vi "tester.vi"() -> ()   [LabVIEW 2014]
uses:
  <vilib>/Utility/inputDevices.llb/closeKeyboard.vi
  <vilib>/Utility/inputDevices.llb/keyboardAcquire.vi
panel:
  in  "stop":bool
  in  "SnakeLeght":i32=5
  out "Real 2D Array":u32[][](array[numeric])
  in  "FieldSizeY":i32=15
  in  "FieldSizeX":i32=10
  out "SnakeWorld":bool[][](array[boolean])
  in  "StartPointY":i32=5
  in  "StartPointX":i32=5
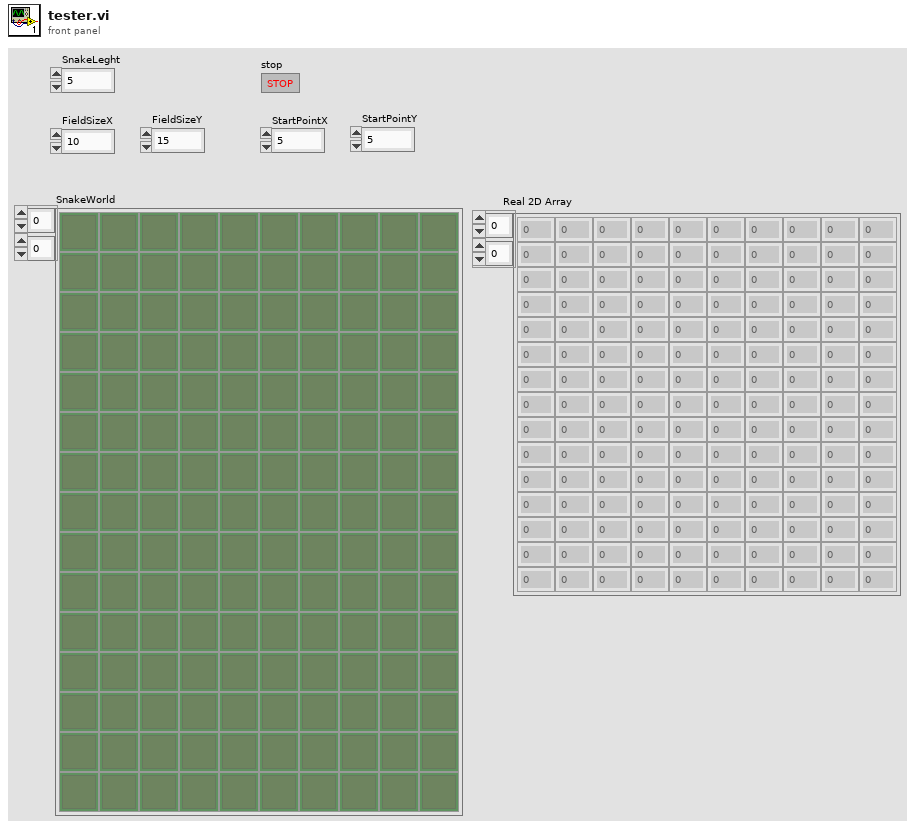
[diagram p1: front panel]
types:
  T1 = enum16{"0", "1", "2", "3", "4", "5", "6", "7", "8", "9", "A", "B", "C", "D", "E", "F", "G", "H", "I", "J", "K", "L", "M", "N", "O", "P", "Q", "R", "S", "T", "U", "V", "W", "X", "Y", "Z", "F1", "F2", "F3", "F4", "F5", "F6", "F7", "F8", "F9", "F10", "F11", "F12", "F13", "F14", "F15", "ADD", "BACK", "BACKSLASH", "CAPITAL", "COMMA", "DECIMAL", "DELETE", "DIVIDE", "DOWN", "END", "EQUALS", "ESCAPE", "GRAVE (`)", "HOME", "INSERT", "LBRACKET", "LCONTROL", "LEFT", "L ALT", "LSHIFT", "LWIN", "MINUS", "MULTIPLY", "NEXT", "NUMLOCK", "NUMPAD_0", "NUMPAD_1", "NUMPAD_2", "NUMPAD_3", "NUMPAD_4", "NUMPAD_5", "NUMPAD_6", "NUMPAD_7", "NUMPAD_8", "NUMPAD_9", "PAUSE", "PERIOD", "PRIOR (PG UP)", "RBRACKET", "RCONTROL", "RETURN", "RIGHT", "R ALT", "RSHIFT", "RWIN", "SCROLL", "SEMICOLON", "SLASH", "SPACE", "SUBTRACT", "TAB", "UP", "ENTER (num pad)", "' (quote)"}
  T2 = enum16{"0", "1", "2", "3", "4", "5", "6", "7", "8", "9", "A", "B", "C", "D", "E", "F", "G", "H", "I", "J", "K", "L", "M", "N", "O", "P", "Q", "R", "S", "T", "U", "V", "W", "X", "Y", "Z", "F1", "F2", "F3", "F4", "F5", "F6", "F7", "F8", "F9", "F10", "F11", "F12", "F13", "F14", "F15", "ADD", "BACK", "BACKSLASH", "CAPITAL", "COMMA", "DECIMAL", "DELETE", "DIVIDE", "DOWN", "END", "EQUALS", "ESCAPE", "GRAVE (`)", "HOME", "INSERT", "LBRACKET", "LCONTROL", "LEFT", "L ALT", "LSHIFT", "LWIN", "MINUS", "MULTIPLY", "NEXT", "NUMLOCK", "NUMPAD_0", "NUMPAD_1", "NUMPAD_2", "NUMPAD_3", "NUMPAD_4", "NUMPAD_5", "NUMPAD_6", "NUMPAD_7", "NUMPAD_8", "NUMPAD_9", "PAUSE", "PERIOD", "PRIOR (PG UP)", "RBRACKET", "RCONTROL", "RETURN", "RIGHT", "R ALT", "RSHIFT", "RWIN", "SCROLL", "SEMICOLON", "SLASH", "SPACE", "SUBTRACT", "TAB", "UP", "ENTER (num pad)", "' (quote)"}[]
  T3 = typedef "SnakeMovements.ctl" = enum16{"STOP", "UP", "DOWN", "RIGHT", "LEFT"}
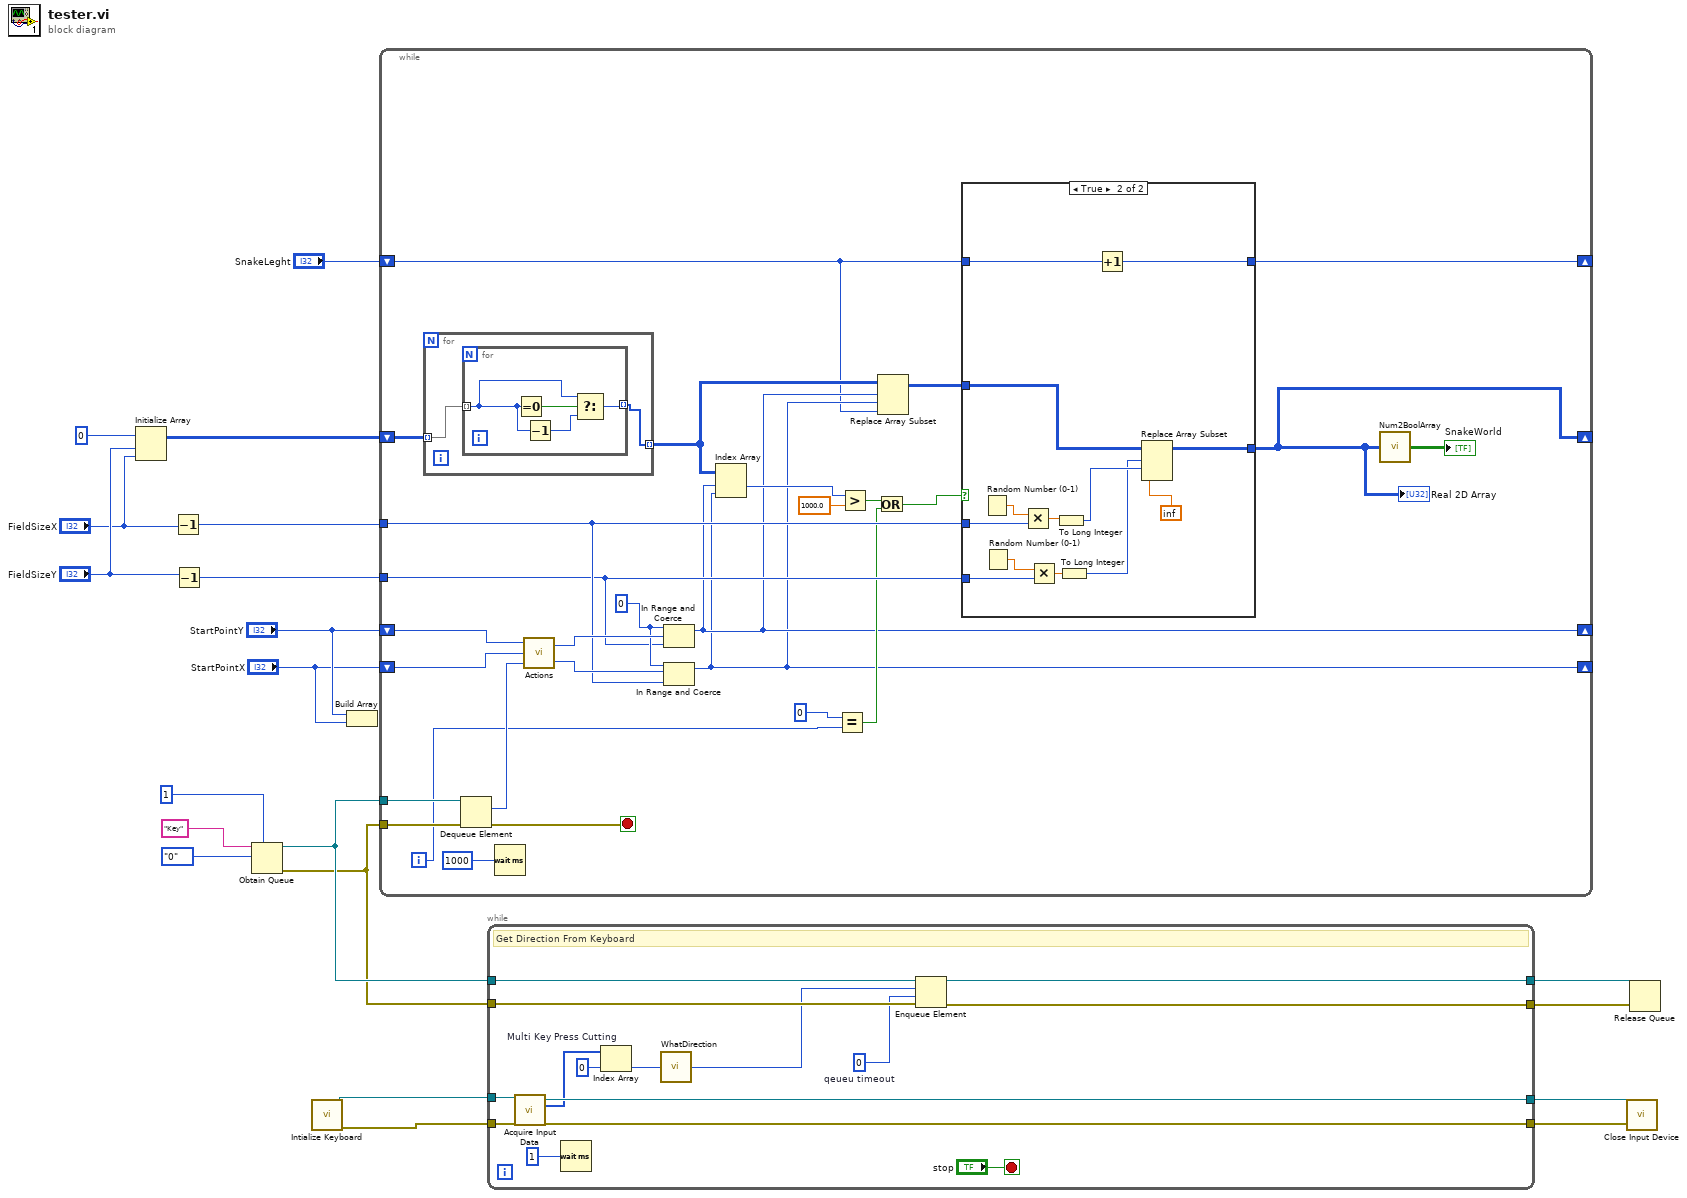
[diagram p0: block diagram]
diagram:
  n1 = Initialize Array(0, "FieldSizeY", "FieldSizeX") -> (w1:i32[][])
  n2 = Decrement(x="FieldSizeX") -> (x-1=w7:i32)
  n3 = Decrement(x="FieldSizeY") -> (x-1=w8:i32)
  n4 = Obtain Queue(max queue size (-1, unlimited)=1, name (unnamed)="Key", element data type=T1."0" ("element")) -> (queue out=w13:refnum<queue>, error out=w12:errorcluster)  [unwired: 2 in, 1 out]
  n5 = call <vilib>:"Intialize Keyboard.vi"() -> ("error out"=w19:errorcluster, "device ID"=w20:refnum<k1>)  [unwired: 10 in]
  n6 = Build Array("StartPointY", "StartPointX") -> ()  [unwired: 1 out]
  n7 = while {
    shift-right: [w24] -> _
    shift-left: "StartPointY" -> [w43]
    shift-right: [w23] -> _
    shift-left: "StartPointX" -> [w44]
    tunnel: w13 -> [w47]
    tunnel: w12 -> [w46]
    tunnel: w8 -> [w35]
    tunnel: w7 -> [w36]
    shift-right: [w34] -> _
    shift-left: w1 -> [w37]
    shift-right: [w22] -> _
    shift-left: "SnakeLeght" -> [w21]
    i -> [w30]
    stop <- w38 stop-if-true
    w40 = 0 ("upper limit")
    n8 = for {
      tunnel: w37 -> [w65] mode=indexing
      tunnel: [w64] -> w31 mode=indexing
      n9 = for {
        tunnel: w65 -> [w66] mode=indexing
        tunnel: [w68] -> w64 mode=indexing
        n10 = Equal To 0?(x=w66) -> (x = 0?=w69:bool)
        n11 = Decrement(x=w66) -> (x-1=w67:i32)
        n12 = Select(t=w66, s=w69, f=w67) -> (s? t:f=w68:i32)
      }
    }
    n13 = Dequeue Element(queue=w47, error in (no error)=w46) -> (element=w45:T1, error out=w38:errorcluster)  [unwired: 1 in, 2 out]
    n14 = Wait (ms)(milliseconds to wait=u32 1000) -> ()  [unwired: 1 out]
    n15 = call "Actions.vi"("direction"=w45, "X coordinate IN"=w44, "Y coordinate IN"=w43) -> ("X coordinate OUT"=w41:i32, "Y coordinate OUT"=w42:i32)
    n16 = In Range and Coerce(upper limit=w40, x=w42, lower limit=w35) -> (coerced(x)=w24:i32)  [unwired: 1 out]
    n17 = In Range and Coerce(upper limit=w40, x=w41, lower limit=w36) -> (coerced(x)=w23:i32)  [unwired: 1 out]
    n18 = Index Array(array=w31, index (row)=w24, index (col)=w23) -> (element=w28:i32)
    n19 = Equal?(x=0, y=w30) -> (x = y?=w27:bool)
    n20 = Greater?(x=w28, y=1000.0) -> (0:w26:bool)
    n21 = Or(x=w26, y=w27) -> (x .or. y?=w25:bool)
    n22 = Replace Array Subset(array=w31, new element=w21, index (row)=w24, index (col)=w23) -> (w33:i32[][])
    n23 = case shown="True" w25 {
      tunnel: w36 -> [_ w61]
      tunnel: w35 -> [_ w60]
      tunnel: [w50 w57] -> w34
      tunnel: w33 -> [w50 w56]
      tunnel: [w49 w51] -> w22
      tunnel: w21 -> [w49 w52]
      frame False {
      }
      frame True {
        n24 = Random Number (0-1)() -> (number: 0 to 1=w63:dbl)
        n25 = Random Number (0-1)() -> (number: 0 to 1=w62:dbl)
        n26 = Multiply(x=w63, y=w61) -> (x*y=w59:dbl)
        n27 = Multiply(x=w62, y=w60) -> (x*y=w58:dbl)
        n28 = To Long Integer(number=w59) -> (32bit integer=w55:i32)
        n29 = To Long Integer(number=w58) -> (32bit integer=w54:i32)
        n30 = Increment(x=w52) -> (x+1=w51:i32)
        n31 = Replace Array Subset(array=w56, new element=inf, index (row)=w54, index (col)=w55) -> (w57:i32[][])
      }
    }
    "Real 2D Array" <- w34
    n32 = call "Num2BoolArray.vi"("Real 2D Array"=w34) -> ("BooleanArray"=→"SnakeWorld":bool[][])
  }
  n33 = while {
    tunnel: w20 -> [w84]
    tunnel: w19 -> [w83]
    tunnel: [w82] -> w18
    tunnel: [w81] -> w17
    tunnel: w12 -> [w75]
    tunnel: w13 -> [w76]
    tunnel: [w73] -> w11
    tunnel: [w72] -> w10
    stop <- "stop" stop-if-true
    w71 = 0  # qeueu timeout
    # "Get Direction From Keyboard"
    n34 = call-poly <vilib>:"Acquire Input Data.vi"("device ID"=w84, "error in (no error)"=w83) -> ("device ID"=w82:refnum<k1>, "keys pressed"=w79:T2, "error out"=w81:errorcluster)  [unwired: 15 in]
    n35 = Wait (ms)(milliseconds to wait=u32 1) -> ()  [unwired: 1 out]
    n36 = Index Array "Multi Key Press Cutting"(array=w79, index=0) -> (element=w77:T1)
    n37 = call "WhatDirection.vi"("key"=w77) -> ("Movement"=w74:T3)
    n38 = Enqueue Element(queue=w76, element=w74, timeout in ms (-1)=w71, error in (no error)=w75) -> (queue out=w73:refnum<queue>, error out=w72:errorcluster)  [unwired: 1 out]
  }
  n39 = call-poly <vilib>:"Close Input Device.vi"("error in (no error)"=w17, "device ID"=w18) -> ()  [unwired: 8 in, 1 out]
  n40 = Release Queue(queue=w11, error in (no error)=w10) -> ()  [unwired: 1 in, 3 out]
